vi "Read UDP.vi"(11 "String":string) -> (2 "2 Point":dbl, 3 "3 Point":dbl)   [LabVIEW 2012]
panel:
  out "Array":dbl[](array[numeric])
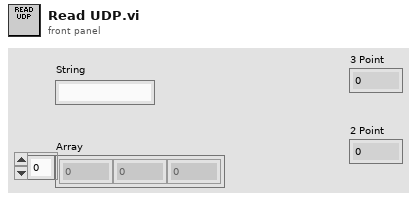
[diagram p1: front panel]
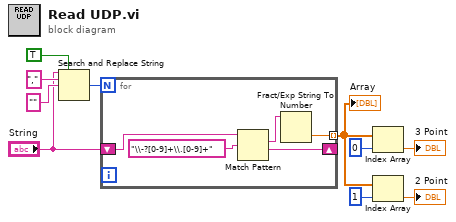
[diagram p0: block diagram]
diagram:
  n1 = Search and Replace String(replace all?=TRUE ("replace all? (F)"), input string="String", search string="," ("substring (\"\")"), replace string="" ("replace string (\"\")")) -> (number of replacements=w1:i32)  [unwired: 4 in, 3 out]
  n2 = for {
    N: w1 -> [_]
    shift-right: [w13] -> _
    shift-left: "String" -> [w14]
    tunnel: [w11] -> w4 mode=indexing
    n3 = Match Pattern(string=w14, regular expression="\\-?[0-9]+\\.[0-9]+") -> (match substring=w12:string, after substring=w13:string)  [unwired: 1 in, 2 out]
    n4 = Fract/Exp String To Number(string=w12) -> (number=w11:dbl)  [unwired: 3 in, 1 out]
  }
  "Array" <- w4
  n5 = Index Array(array=w4, index=0) -> (element=→"3 Point":dbl)
  n6 = Index Array(array=w4, index=1) -> (element=→"2 Point":dbl)
